vi "19_1.vi"() -> ()   [LabVIEW 2018]
uses:
  <userlib>/_OpenG.lib/array/array.llb/Search 1D Array (String)__ogtk.vi
  <userlib>/_OpenG.lib/array/array.llb/Delete Elements from 1D Array (String)__ogtk.vi
panel:
  out "size(s)":i32
  out "Rule 0":string[](array[string])
  out "Array":cluster{string[][]}[](array[cluster])
  out "Decoded Rules":cluster{string[][]}[](array[cluster])
  out "Rules":string[](array[string])
  out "Messages":string[](array[string])
  in  "Input":string
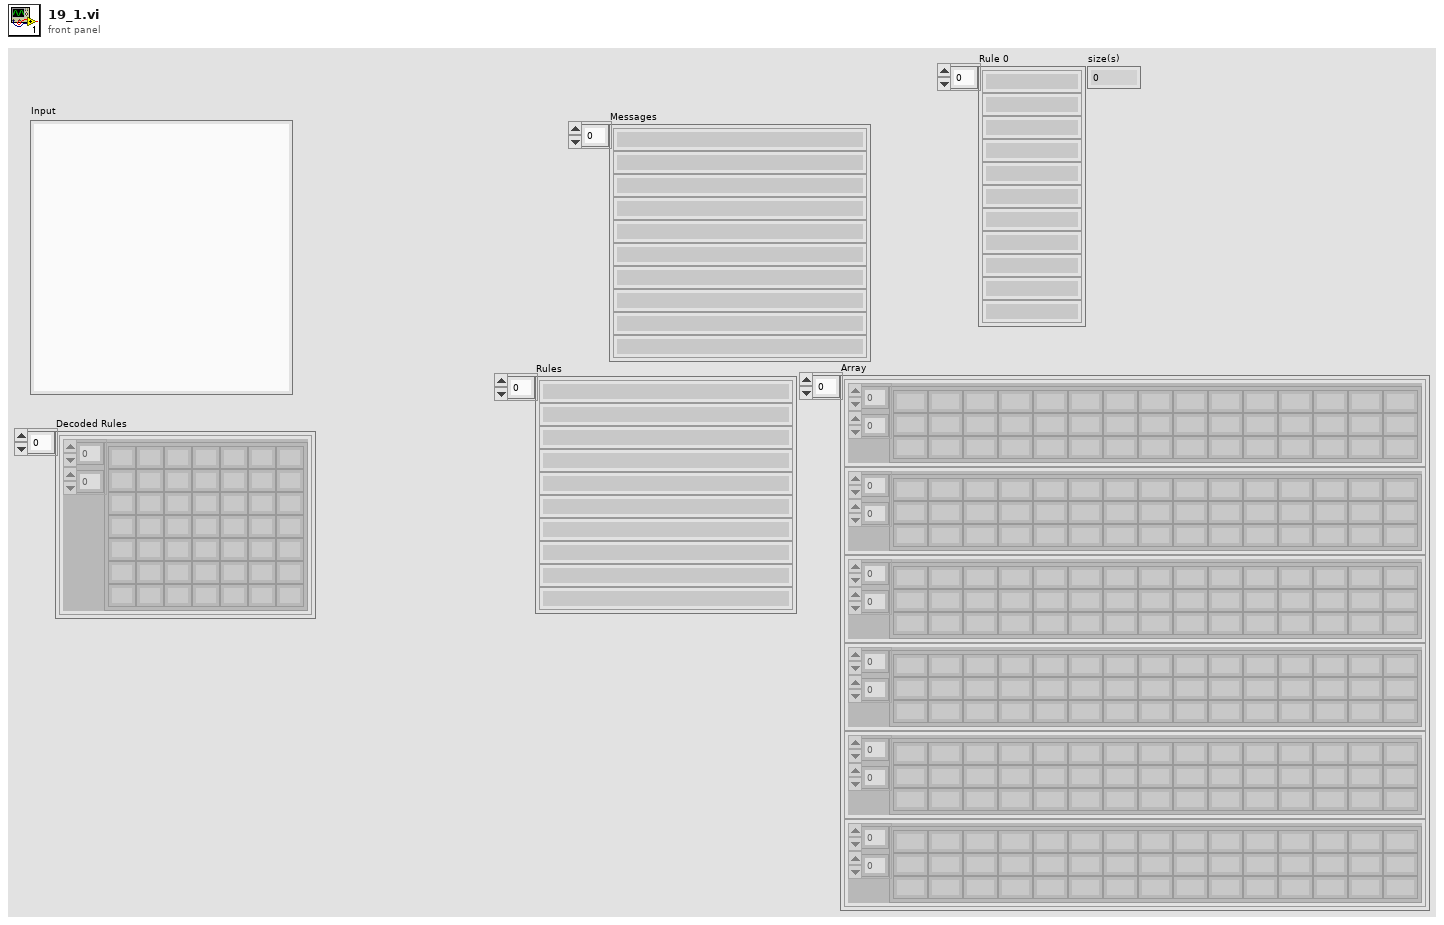
[diagram p1: front panel]
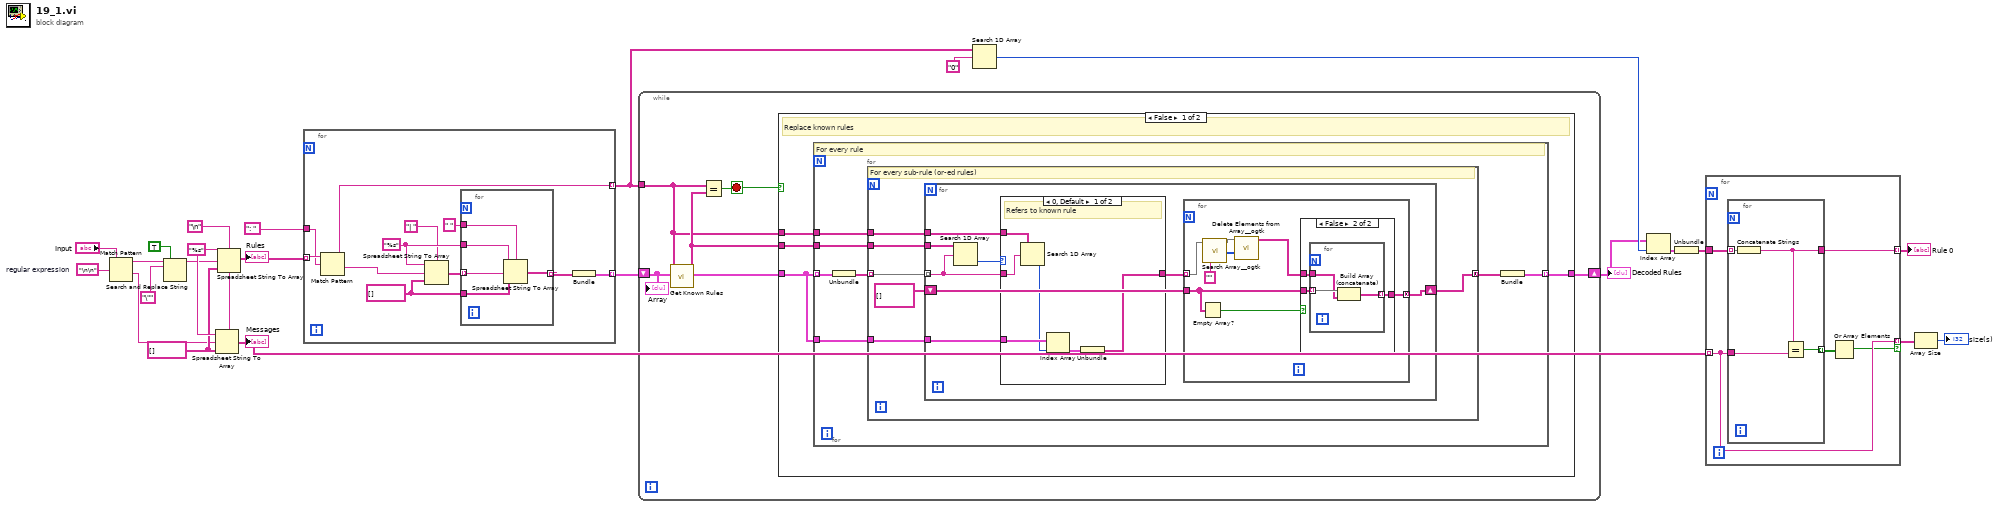
[diagram p0: block diagram]
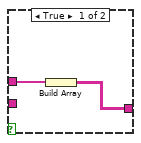
[diagram p2: hidden frame]
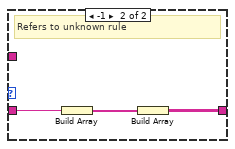
[diagram p3: hidden frame]
diagram:
  w19 = "\n"
  w21 = "%s"
  w20 = string[] []
  w22 = "\n\n"  # regular expression
  n1 = Match Pattern(string="Input", regular expression=w22) -> (before substring=w15:string, after substring=w16:string)  [unwired: 1 in, 2 out]
  n2 = Search and Replace String(replace all?=TRUE ("replace all? (F)"), input string=w15, search string="\"") -> (result string=w14:string)  [unwired: 5 in, 3 out]
  n3 = Spreadsheet String To Array(delimiter (Tab)=w19, format string=w21, spreadsheet string=w16, array type (2D Dbl)=w20) -> (array=w3:string[])
  "Messages" <- w3
  n4 = Spreadsheet String To Array(delimiter (Tab)=w19, format string=w21, spreadsheet string=w14, array type (2D Dbl)=w20) -> (array=w18:string[])
  "Rules" <- w18
  n5 = for {
    tunnel: w18 -> [w27] mode=indexing
    tunnel: ": " -> [w24]
    tunnel: [w26] -> w10 mode=indexing
    tunnel: [w29] -> w11 mode=indexing
    w33 = "%s"
    w32 = string[] []
    n6 = Match Pattern(string=w27, regular expression=w24) -> (before substring=w26:string, after substring=w25:string)  [unwired: 1 in, 2 out]
    n7 = Spreadsheet String To Array(delimiter (Tab)="| ", format string=w33, spreadsheet string=w25, array type (2D Dbl)=w32) -> (array=w34:string[])
    n8 = for {
      tunnel: w34 -> [w39] mode=indexing
      tunnel: w33 -> [w38]
      tunnel: w32 -> [w37]
      tunnel: " " -> [w36]
      tunnel: [w35] -> w28 mode=indexing
      n9 = Spreadsheet String To Array(delimiter (Tab)=w36, format string=w38, spreadsheet string=w39, array type (2D Dbl)=w37) -> (array=w35:string[])
    }
    n10 = Bundle(w28) -> (w29:cluster{string[][]})  [unwired: 1 in]
  }
  n11 = while {
    tunnel: w10 -> [w40]
    shift-right: [w42] -> w7
    shift-left: w11 -> [w43]
    stop <- w44 stop-if-true
    n12 = call "Get Known Rules.vi"("Rules"=w43, "Rule ID's"=w40) -> ("Known Rules"=w41:string[])  [unwired: 9 in]
    n13 = Equal?(x=w40, y=w41) -> (x = y?=w44:bool)
    n14 = case shown="False" w44 {
      tunnel: w43 -> [w45 w94]
      tunnel: [w47 w94] -> w42
      tunnel: w41 -> [w48 _]
      tunnel: w40 -> [w46 _]
      frame False {
        # "Replace known rules"
        n15 = for {
          tunnel: w45 -> [w55] mode=indexing
          tunnel: w48 -> [w52]
          tunnel: [w53] -> w47 mode=indexing
          tunnel: w46 -> [w51]
          tunnel: w45 -> [w50]
          # "For every rule"
          n16 = Unbundle(w55) -> (w49:string[][])
          n17 = for {
            tunnel: w49 -> [w61] mode=indexing
            tunnel: [w56] -> w54 mode=concatenating
            tunnel: w52 -> [w60]
            tunnel: w51 -> [w59]
            tunnel: w50 -> [w58]
            # "For every sub-rule (or-ed rules)"
            n18 = for {
              tunnel: w61 -> [w67] mode=indexing
              tunnel: w60 -> [w69]
              tunnel: w59 -> [w66]
              tunnel: w58 -> [w65]
              shift-right: [w62] -> w56
              shift-left: string[][] [] -> [w63]
              n19 = Search 1D Array(1D array=w69, element=w67) -> (index of element=w68:i32)  [unwired: 1 in]
              n20 = case shown="0, Default" w68 {
                tunnel: w67 -> [w89 w93]
                tunnel: [w85 w91] -> w64
                tunnel: w66 -> [w90 _]
                tunnel: w65 -> [w88 _]
                frame 0, Default {
                  # "Refers to known rule"
                  n21 = Search 1D Array(1D array=w90, element=w89) -> (index of element=w87:i32)  [unwired: 1 in]
                  n22 = Index Array(array=w88, index=w87) -> (element=w86:cluster{string[][]})
                  n23 = Unbundle(w86) -> (w85:string[][])
                }
                frame -1 {
                  # "Refers to unknown rule"
                  n24 = Build Array(w93) -> (w92:string[])
                  n25 = Build Array(w92) -> (w91:string[][])
                }
              }
              n26 = for {
                tunnel: w64 -> [w71] mode=indexing
                tunnel: w63 -> [w75]
                tunnel: [w76] -> w62 mode=concatenating
                n27 = Empty Array?(array=w75) -> (empty?=w74:bool)
                n28 = call-poly <userlib>:"Search Array__ogtk.vi"("Array"=w71, "Element Data"="") -> ("Indices of Elements"=w73:i32[])  [unwired: 7 in]
                n29 = call-poly <userlib>:"Delete Elements from Array__ogtk.vi"("indices"=w73, "array"=w71) -> ("array w/ subset deleted"=w72:string[])  [unwired: 8 in, 1 out]
                n30 = case shown="False" w74 {
                  tunnel: w72 -> [w78 w81]
                  tunnel: [w77 w80] -> w76
                  tunnel: w75 -> [_ w79]
                  frame True {
                    n31 = Build Array(w78) -> (w77:string[][])
                  }
                  frame False {
                    n32 = for {
                      tunnel: w79 -> [w84] mode=indexing
                      tunnel: w81 -> [w83]
                      tunnel: [w82] -> w80 mode=indexing
                      n33 = Build Array (concatenate)(w84, w83) -> (w82:string[])
                    }
                  }
                }
              }
            }
          }
          n34 = Bundle(w54) -> (w53:cluster{string[][]})  [unwired: 1 in]
        }
      }
      frame True {
        # "All Rules are known"
      }
    }
    "Array" <- w43
  }
  "Decoded Rules" <- w7
  n35 = Search 1D Array(1D array=w10, element="0") -> (index of element=w8:i32)  [unwired: 1 in]
  n36 = Index Array(array=w7, index=w8) -> (element=w6:cluster{string[][]})
  n37 = Unbundle(w6) -> (w5:string[][])
  n38 = for {
    tunnel: w5 -> [w99]
    tunnel: [w98] -> w4 mode=indexing
    tunnel: w3 -> [w96] mode=indexing
    tunnel: [w96] -> w2 mode=indexing if=w95
    n39 = for {
      tunnel: w99 -> [w103] mode=indexing
      tunnel: [w101] -> w98
      tunnel: w96 -> [w102]
      tunnel: [w100] -> w97 mode=indexing
      n40 = Concatenate Strings(w103) -> (w101:string)
      n41 = Equal?(x=w101, y=w102) -> (x = y?=w100:bool)
    }
    n42 = Or Array Elements(Boolean array=w97) -> (logical OR=w95:bool)
  }
  "Rule 0" <- w4
  n43 = Array Size(array=w2) -> (size(s)=→"size(s)":i32)
